vi "SDGiiControlLoop.vi"(8 "queue error in":errorcluster, 10 "VISA resource":refnum<visa-resource-name>, 11 "queue in":refnum<queue>) -> (0 "error out":errorcluster, 3 "queue out":refnum<queue>)   [LabVIEW 2012]
uses:
  Laser_Status.ctl
  <userlib>/Utility/ErrorLog_lib.lvlib
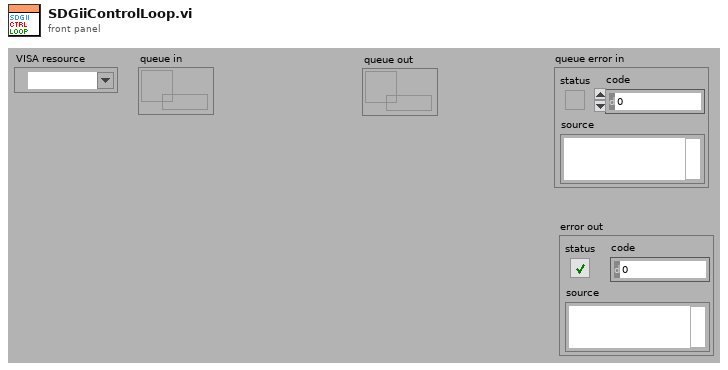
[diagram p1: front panel]
types:
  T1 = typedef "Laser_Status.ctl" = cluster{"State":enum16{"Initialize", "Idle/Update", "Configure", "Turn On", "Tun OFF", "Continuous", "Single Shot", "ManualTrigger", "Close", "Quit"}, "Parameter":dbl}
  T2 = enum16{"Initialize", "Write", "Write/Read", "Read", "Clear", "Close"}
  T3 = enum16{"Initialize", "Idle/Update", "Configure", "Turn On", "Tun OFF", "Continuous", "Single Shot", "ManualTrigger", "Close", "Quit"}
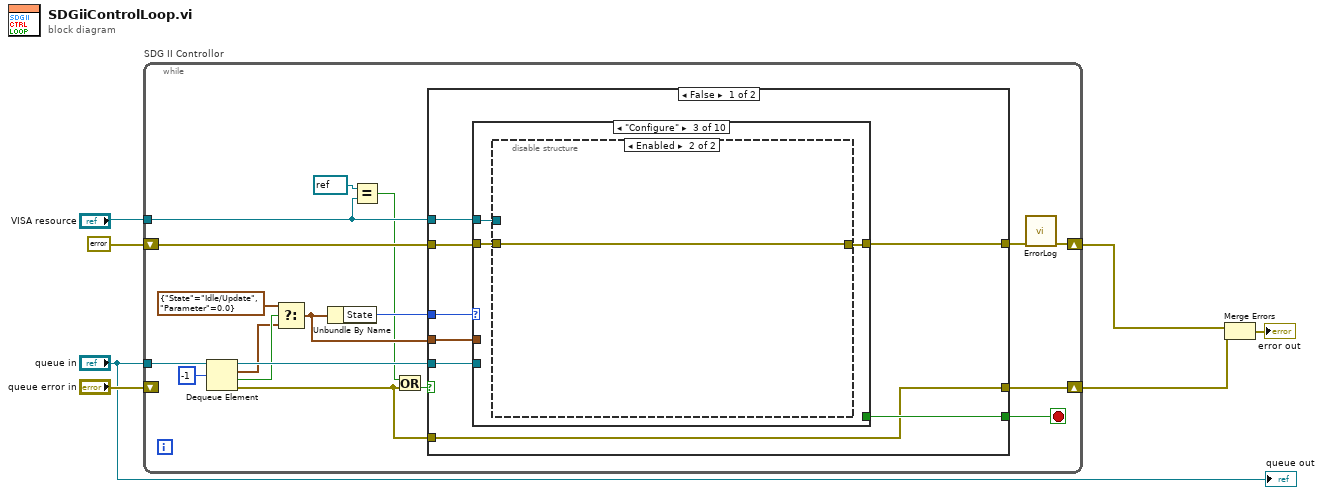
[diagram p0: block diagram]
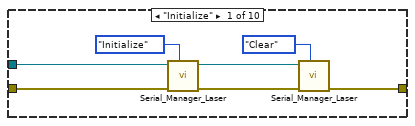
[diagram p2: hidden frame]
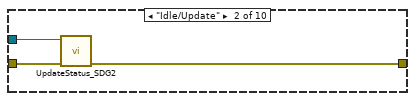
[diagram p3: hidden frame]
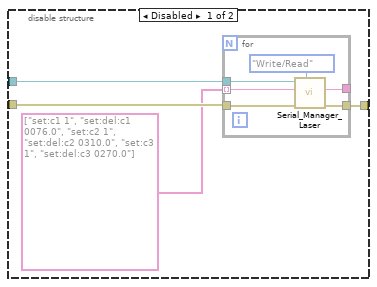
[diagram p4: hidden frame]
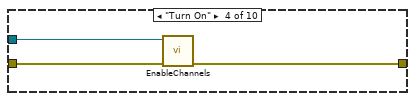
[diagram p5: hidden frame]
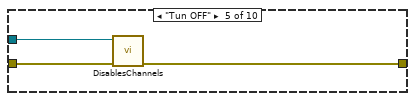
[diagram p6: hidden frame]
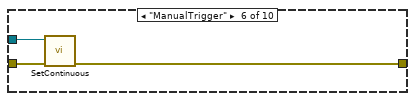
[diagram p7: hidden frame]
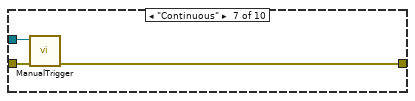
[diagram p8: hidden frame]
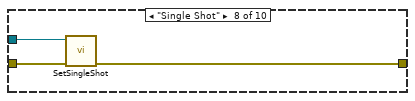
[diagram p9: hidden frame]
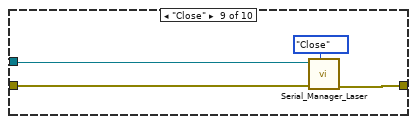
[diagram p10: hidden frame]
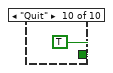
[diagram p11: hidden frame]
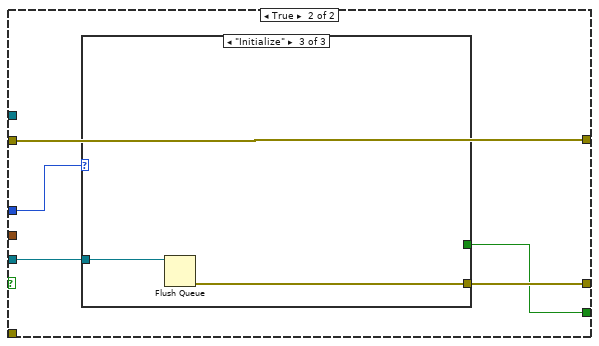
[diagram p12: hidden frame]
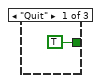
[diagram p13: hidden frame]
diagram:
  n1 = while "SDG II Controllor" {
    tunnel: "queue in" -> [w25]
    shift-right: [w13] -> w2
    shift-left: errorcluster {"status"=FALSE, "code"=0, "source"=""} ("error out") -> [w15]
    shift-right: [w23] -> w3
    shift-left: "queue error in" -> [_]
    tunnel: "VISA resource" -> [w11]
    stop <- w14 stop-if-true
    n2 = Dequeue Element(queue=w25, timeout in ms (-1)=-1) -> (queue out=w24:refnum<queue>, element=w17:T1, timed out?=w21:bool, error out=w8:errorcluster)  [unwired: 1 in]
    n3 = Select(t=T1 {"State"=enum."Idle/Update", "Parameter"=0.0} ("Idle"), s=w21, f=w17) -> (s? t:f=w18:T1)
    n4 = Unbundle By Name(w18) -> ("State"=w19:T3)
    n5 = Equal?(x=refnum<visa-resource-name> refnum ("VISA resource"), y=w11) -> (x = y?=w9:bool)
    n6 = Or(x=w9, y=w8) -> (x .or. y?=w10:bool)
    n7 = case shown="False" w10 {
      tunnel: w19 -> [w33 w78]
      tunnel: w15 -> [w29 w81]
      tunnel: w24 -> [w32 w80]
      tunnel: [w26 w79] -> w23
      tunnel: [w27 w81] -> w22
      tunnel: w18 -> [w30 _]
      tunnel: w11 -> [w31 _]
      tunnel: [w28 w77] -> w14
      tunnel: w8 -> [w26 _]
      frame False {
        n8 = case shown="\"Configure\"" w33 {
          tunnel: w29 -> [w39 w41 w45 w58 w62 w65 w67 w70 w74 _]
          tunnel: w32 -> [_ _ _ _ _ _ _ _ _ _]
          tunnel: w31 -> [w37 w42 w43 w59 w61 w64 w68 w71 w72 _]
          tunnel: [w38 w40 w44 w57 w60 w63 w66 w69 w73 _] -> w27
          tunnel: w30 -> [_ _ _ _ _ _ _ _ _ _]
          tunnel: [_ _ _ _ _ _ _ _ _ TRUE] -> w28
          frame "Initialize" {
            n9 = call "Serial_Manager_Laser.vi"("Job"=T2."Initialize", "error in"=w39, "VISA resource"=w37) -> ("error out"=w34:errorcluster)  [unwired: 7 in, 1 out]
            n10 = call "Serial_Manager_Laser.vi"("Job"=T2."Clear", "error in"=w34, "VISA resource"=w37) -> ("error out"=w38:errorcluster)  [unwired: 7 in, 1 out]
          }
          frame "Idle/Update" {
            n11 = call "UpdateStatus_SDG2.vi"("error in"=w41, "VISA resource"=w42) -> ("error out"=w40:errorcluster)  [unwired: 8 in]
          }
          frame "Configure" {
            n12 = disable-structure shown="Enabled" {
              disable-tunnel: w45 -> [w49 w56]
              disable-tunnel: [w48 w56] -> w44
              disable-tunnel: w43 -> [w47 _]
              frame Disabled {
                n13 = for {
                  tunnel: w49 -> [w54]
                  tunnel: [w53] -> w48
                  tunnel: w47 -> [w52]
                  tunnel: string[] ["set:c1 1", "set:del:c1 0076.0", "set:c2 1", "set:del:c2 0310.0", "set:c3 1", "set:del:c3 0270.0"] -> [w51] mode=indexing
                  tunnel: [w50] -> _
                  n14 = call "Serial_Manager_Laser.vi"("Job"=T2."Write/Read", "error in"=w54, "write buffer"=w51, "VISA resource"=w52) -> ("error out"=w53:errorcluster, "read buffer"=w50:string)  [unwired: 6 in]
                }
              }
              frame Enabled {
              }
            }
          }
          frame "Turn On" {
            n15 = call "EnableChannels.vi"("error in"=w58, "VISA resource"=w59) -> ("error out"=w57:errorcluster)  [unwired: 9 in]
          }
          frame "Tun OFF" {
            n16 = call "DisablesChannels.vi"("error in"=w62, "VISA resource"=w61) -> ("error out"=w60:errorcluster)  [unwired: 9 in]
          }
          frame "ManualTrigger" {
            n17 = call "SetContinuous.vi"("error in"=w65, "VISA resource"=w64) -> ("error out"=w63:errorcluster)  [unwired: 9 in]
          }
          frame "Continuous" {
            n18 = call "ManualTrigger.vi"("error in"=w67, "VISA resource"=w68) -> ("error out"=w66:errorcluster)  [unwired: 9 in]
          }
          frame "Single Shot" {
            n19 = call "SetSingleShot.vi"("error in"=w70, "VISA resource"=w71) -> ("error out"=w69:errorcluster)  [unwired: 9 in]
          }
          frame "Close" {
            n20 = call "Serial_Manager_Laser.vi"("Job"=T2."Close", "error in"=w74, "VISA resource"=w72) -> ("error out"=w73:errorcluster)  [unwired: 7 in, 1 out]
          }
          frame "Quit" {
          }
        }
      }
      frame True {
        n21 = case shown="\"Initialize\"" w78 {
          tunnel: w80 -> [_ _ w84]
          tunnel: [_ _ w83] -> w79
          tunnel: [TRUE _ _] -> w77
          frame "Quit" {
          }
          frame Default {
          }
          frame "Initialize" {
            n22 = Flush Queue(queue=w84) -> (error out=w83:errorcluster)  [unwired: 1 in, 2 out]
          }
        }
      }
    }
    n23 = call <userlib>:"ErrorLog.vi"("error in (no error)"=w22) -> ("error out"=w13:errorcluster)  [unwired: 10 in]
  }
  n24 = Merge Errors(w2, w3) -> (→"error out":errorcluster)
  "queue out" <- "queue in"
